vi "pretv.vi"() -> ()   [LabVIEW 2013]
panel:
  out "Intensity Graph":i16[][](graph)
  in  "Kepfrissites(Hz)":dbl
  out "Sorelterites(Hz)":dbl
  out "Oszolopelterites(Hz)":dbl
  out "Sorelterites":dynamicdata(graph)
  out "Oszolopelterites":dynamicdata(graph)
  in  "stop":bool
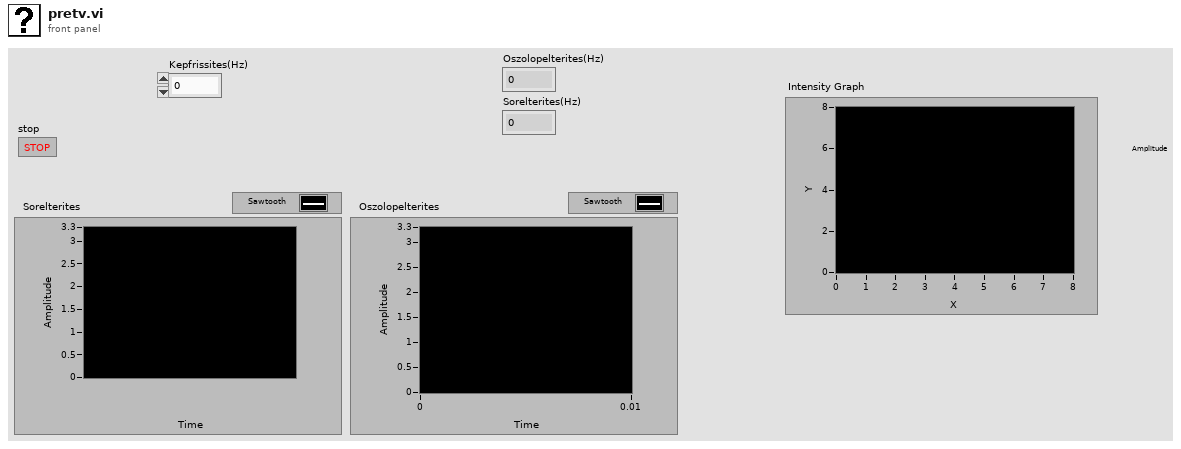
[diagram p1: front panel]
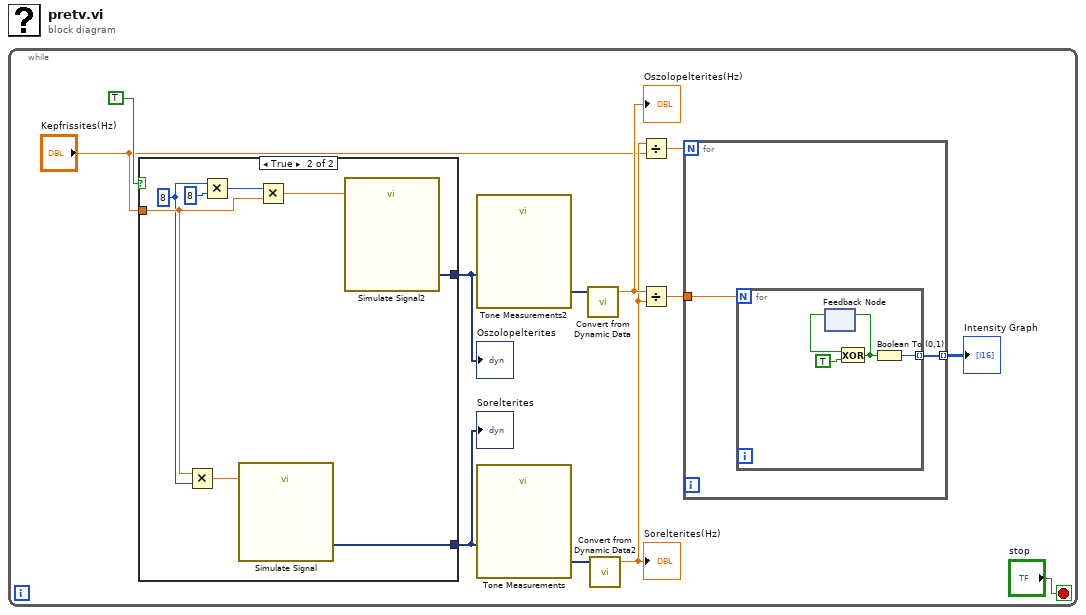
[diagram p0: block diagram]
diagram:
  n1 = while {
    stop <- "stop" stop-if-true
    n2 = case shown="True" TRUE {
      tunnel: [_ w26] -> w11
      tunnel: [_ w25] -> w10
      tunnel: "Kepfrissites(Hz)" -> [_ w20]
      frame False {
      }
      frame True {
        w19 = 8
        n3 = Multiply(x=w20, y=w19) -> (x*y=w24:dbl)
        n4 = Multiply(x=w19, y=8) -> (x*y=w21:i32)
        n5 = call "Simulate Signal"("Frequency"=w24) -> ("Sawtooth"=w26:dynamicdata)  [unwired: 13 in, 1 out]
        n6 = Multiply(x=w21, y=w20) -> (x*y=w23:dbl)
        n7 = call "Simulate Signal2"("Frequency"=w23) -> ("Sawtooth"=w25:dynamicdata)  [unwired: 13 in, 1 out]
      }
    }
    "Oszolopelterites" <- w10
    "Sorelterites" <- w11
    n8 = call "Tone Measurements2"("Signals"=w10) -> ("Frequency"=w8:dynamicdata)  [unwired: 9 in, 1 out]
    n9 = call "Tone Measurements"("Signals"=w11) -> ("Frequency"=w9:dynamicdata)  [unwired: 9 in, 1 out]
    n10 = call "Convert from Dynamic Data"("Dynamic Data Type"=w8) -> ("Scalar"=w6:dbl)  [unwired: 3 in]
    "Oszolopelterites(Hz)" <- w6
    n11 = call "Convert from Dynamic Data2"("Dynamic Data Type"=w9) -> ("Scalar"=w5:dbl)  [unwired: 3 in]
    "Sorelterites(Hz)" <- w5
    n12 = Divide(x=w5, y="Kepfrissites(Hz)") -> (x/y=w2:dbl)
    n13 = Divide(x=w6, y=w5) -> (x/y=w3:dbl)
    n14 = for {
      N: w2 -> [_]
      tunnel: w3 -> [w14]
      tunnel: [w13] -> w1 mode=indexing
      n15 = for {
        N: w14 -> [_]
        tunnel: [w18] -> w13 mode=indexing
        n16 = feedback #1() -> (w16:bool)  [unwired: 1 in]
        n17 = Exclusive Or(1:TRUE ("y"), 2:w16) -> (0:w15:bool)
        n18 = feedback-in #1(w15) -> ()
        n19 = Boolean To (0,1)(Boolean=w15) -> (0, 1=w18:i16)
      }
    }
    "Intensity Graph" <- w1
  }
